vi "Calculate Trigger Wait Cycles.vi"(1 "Frequency (Hz)":dbl, 2 "Period (ms)":dbl) -> (0 "Cycles to Wait":dbl)   [LabVIEW 2013]
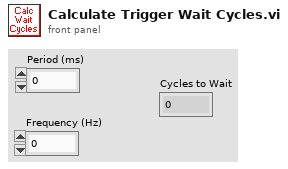
[diagram p1: front panel]
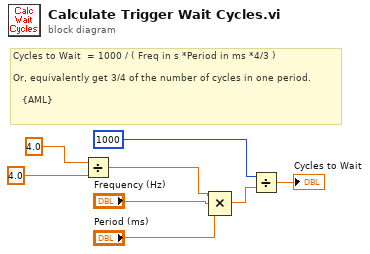
[diagram p0: block diagram]
diagram:
  # "Cycles to Wait  = 1000 / ( Freq in s *Period in ms *4/3 ) \n\nOr, equivalently get 3/4 of the number of cycles in one period.\n\n   {AML}"
  n1 = Divide(x=4.0, y=4.0) -> (x/y=w1:dbl)
  n2 = Compound Arithmetic op=MULTIPLY(w1, "Frequency (Hz)", "Period (ms)") -> (w5:dbl)
  n3 = Divide(x=1000, y=w5) -> (x/y=→"Cycles to Wait":dbl)
